vi "Get Build Name.vi"(7 "error in (no error)":errorcluster, 10 "VISA in":refnum<visa-resource-name>) -> (0 "error out":errorcluster, 2 "Build String":string, 3 "VISA out":refnum<visa-resource-name>)   [LabVIEW 2017, in "Drivers.lvlib" / "ASI TG-1000.lvlib"]
doc: "Tells the ASI controller to move the (single) specified axis to the corresponding specified position; the equivalent of using the MOVE command. Note that it performs no checking to see if the move completes successfully."
uses:
  Utility/Serial Response Syntax.ctl
  ASI TG-1000.lvlib
panel:
  # "NB: the comm port should already be open before using this VI"
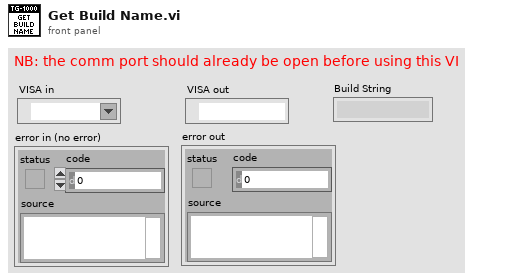
[diagram p1: front panel]
types:
  T1 = typedef "Drivers.lvlib/ASI TG-1000.lvlib/Serial Response Syntax.ctl" = enum16{":A then single line", "Single line, no :A", ":A or : then single line", ":A then single number", ":A or : then single number", ":A then <axis>= single number"}
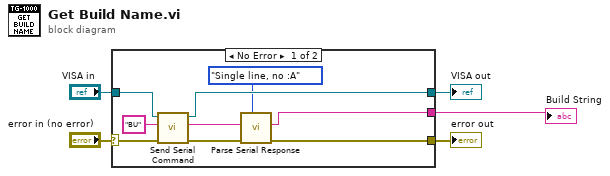
[diagram p0: block diagram]
diagram:
  n1 = case shown="No Error" "error in (no error)" {
    selector: "error in (no error)" -> [w12 w16]
    tunnel: "VISA in" -> [w14 w15]
    tunnel: [w9 w16] -> w3
    tunnel: [w13 w15] -> w2
    tunnel: [w6 _] -> w1
    frame No Error {
      n2 = call "Send Serial Command.vi"("error in (no error)"=w12, "Command"="BU", "VISA in"=w14) -> ("error out"=w10:errorcluster, "Response"=w8:string, "VISA out"=w13:refnum<visa-resource-name>)  [unwired: 6 in]
      n3 = call "Parse Serial Response.vi"("Response Syntax"=Serial_Response_Syntax."Single line, no :A", "error in (no error)"=w10, "Raw Response"=w8) -> ("error out"=w9:errorcluster, "Parsed String"=w6:string)  [unwired: 5 in, 2 out]
    }
    frame Error {
    }
  }
  "VISA out" <- w2
  "error out" <- w3
  "Build String" <- w1
